vi "get file data.vi"(8 "error in":errorcluster, 11 "Path":path) -> (0 "error out":errorcluster, 2 "format":T1)   [LabVIEW 2013, in "NISE_CEF_TreeSerializer.lvlib"]
uses:
  base file format.ctl
  NISE_CEF_TreeSerializer.lvlib
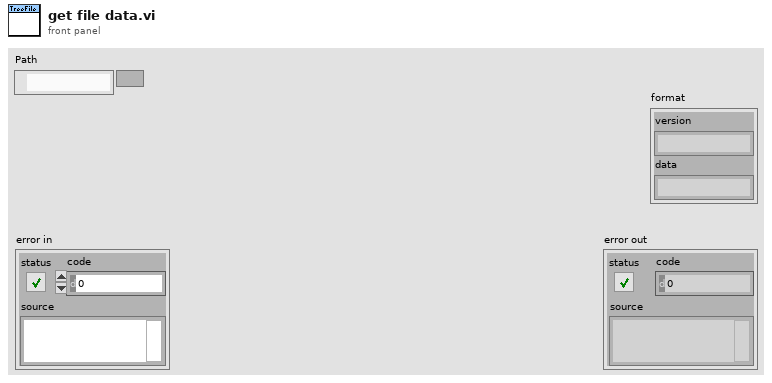
[diagram p1: front panel]
types:
  T1 = typedef "NISE_CEF_TreeSerializer.lvlib/base file format.ctl" = cluster{"version":string, "data":string}
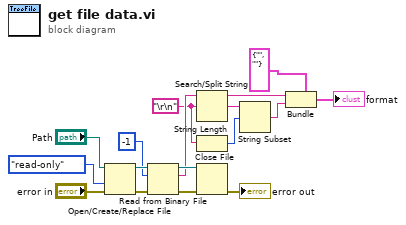
[diagram p0: block diagram]
diagram:
  w4 = "\r\n"
  n1 = Open/Create/Replace File(file path (use dialog)="Path", error in="error in", access (0:read/write)=enum16{"read/write", "read-only", "write-only"}."read-only") -> (refnum out=w11:refnum<file>, error out=w14:errorcluster)  [unwired: 3 in, 1 out]
  n2 = Read from Binary File(8:w14, 10:-1 ("count (1)"), 11:w11) -> (0:w13:errorcluster, 2:w6:string, 3:w10:refnum<file>)  [unwired: 3 in, 1 out]
  n3 = Search/Split String(string=w6, search string/char (-)=w4) -> (substring before match=w5:string, match + rest of string=w2:string)  [unwired: 1 in, 1 out]
  n4 = String Length(string=w4) -> (length=w3:i32)
  n5 = Close File(refnum=w10, error in=w13) -> (error out=→"error out":errorcluster)  [unwired: 1 out]
  n6 = String Subset(string=w2, offset (0)=w3) -> (substring=w1:string)  [unwired: 1 in]
  n7 = Bundle(cluster=T1 {"version"="", "data"=""} ("format"), "version"=w5, "data"=w1) -> (→"format":T1)
